vi "Describe Comparison.vi"(6 "Delta":variant, 9 "Actual":variant, 10 "Expected":variant) -> (2 "Description":string)   [LabVIEW 2020, in "LUnit Test Case.lvclass"]
uses:
  LUnit Test Case.lvclass
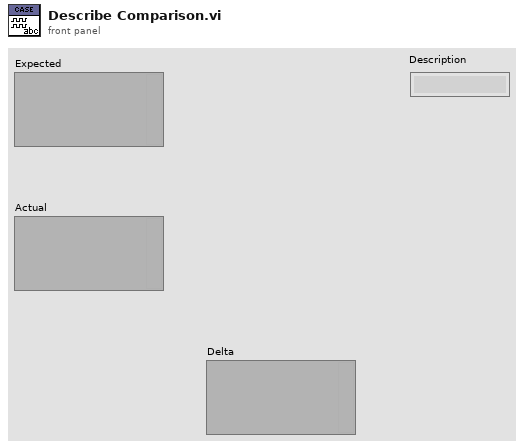
[diagram p1: front panel]
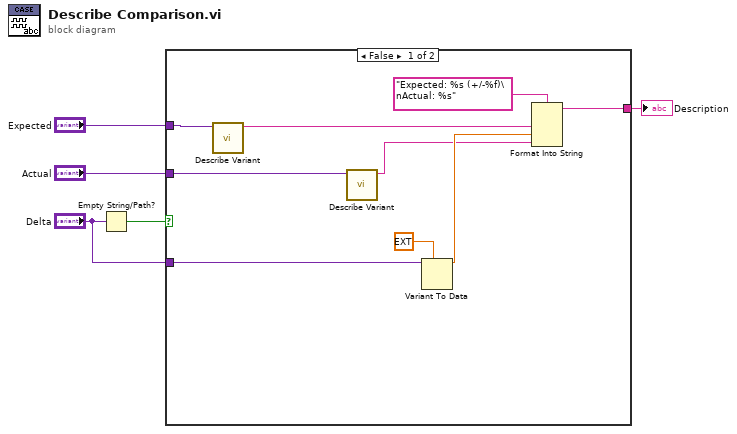
[diagram p0: block diagram]
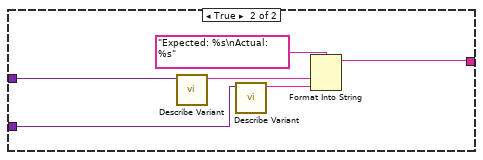
[diagram p2: hidden frame]
diagram:
  n1 = Empty String/Path?(string/path="Delta") -> (empty?=w3:bool)
  n2 = case shown="False" w3 {
    tunnel: "Expected" -> [w11 w17]
    tunnel: "Actual" -> [w9 w16]
    tunnel: "Delta" -> [w10 _]
    tunnel: [w8 w15] -> w1
    frame False {
      n3 = call "Describe Variant.vi"("Variant"=w11) -> ("Variant Description"=w12:string)  [unwired: 8 in, 2 out]
      n4 = call "Describe Variant.vi"("Variant"=w9) -> ("Variant Description"=w6:string)  [unwired: 8 in, 2 out]
      n5 = Variant To Data(type=ext 0.0, Variant=w10) -> (data=w7:ext)  [unwired: 1 in, 1 out]
      n6 = Format Into String(format string="Expected: %s (+/-%f)\nActual: %s", w12, w7, w6) -> (resulting string=w8:string)  [unwired: 2 in, 1 out]
    }
    frame True {
      n7 = call "Describe Variant.vi"("Variant"=w17) -> ("Variant Description"=w20:string)  [unwired: 8 in, 2 out]
      n8 = call "Describe Variant.vi"("Variant"=w16) -> ("Variant Description"=w18:string)  [unwired: 8 in, 2 out]
      n9 = Format Into String(format string="Expected: %s\nActual:   %s", w20, w18) -> (resulting string=w15:string)  [unwired: 2 in, 1 out]
    }
  }
  "Description" <- w1
